vi "Center Scanner Tester.vi"(8 "Hight":u16, 9 "Width":u16, 10 "ImageIn":u8[][](array[numeric]), 11 "StartLine":u32) -> (1 "HorCenter":u16, 3 "ImgOut":u8[][](array[numeric]))   [LabVIEW 2015]
uses:
  <vilib>/Analysis/baseanly.llb/Mean (DBL).vi
  <vilib>/Analysis/NI_AALBase.lvlib
panel:
  out "mean 2":dbl format="%0.2f"
  out "mean":dbl format="%0.2f"
  out "ImageIn 2":u8[][](graph)
  out "ImgOut 2":u8[][](graph)
  out "max index(es) 2":i32
  out "element 2":dbl
  out "element":dbl
  out "max index(es)":i32
  out "size(s) 2":i32
  out "size(s)":i32
  out "Histogram Graph 2":T1(graph)
  out "Histogram Graph":T1(graph)
  out "Radiuses 2":i32[](graph)
  out "Centers 2":i32[](graph)
  out "Radiuses":i32[](graph)
  out "Centers":i32[](graph)
  in  "Delta":u32=2
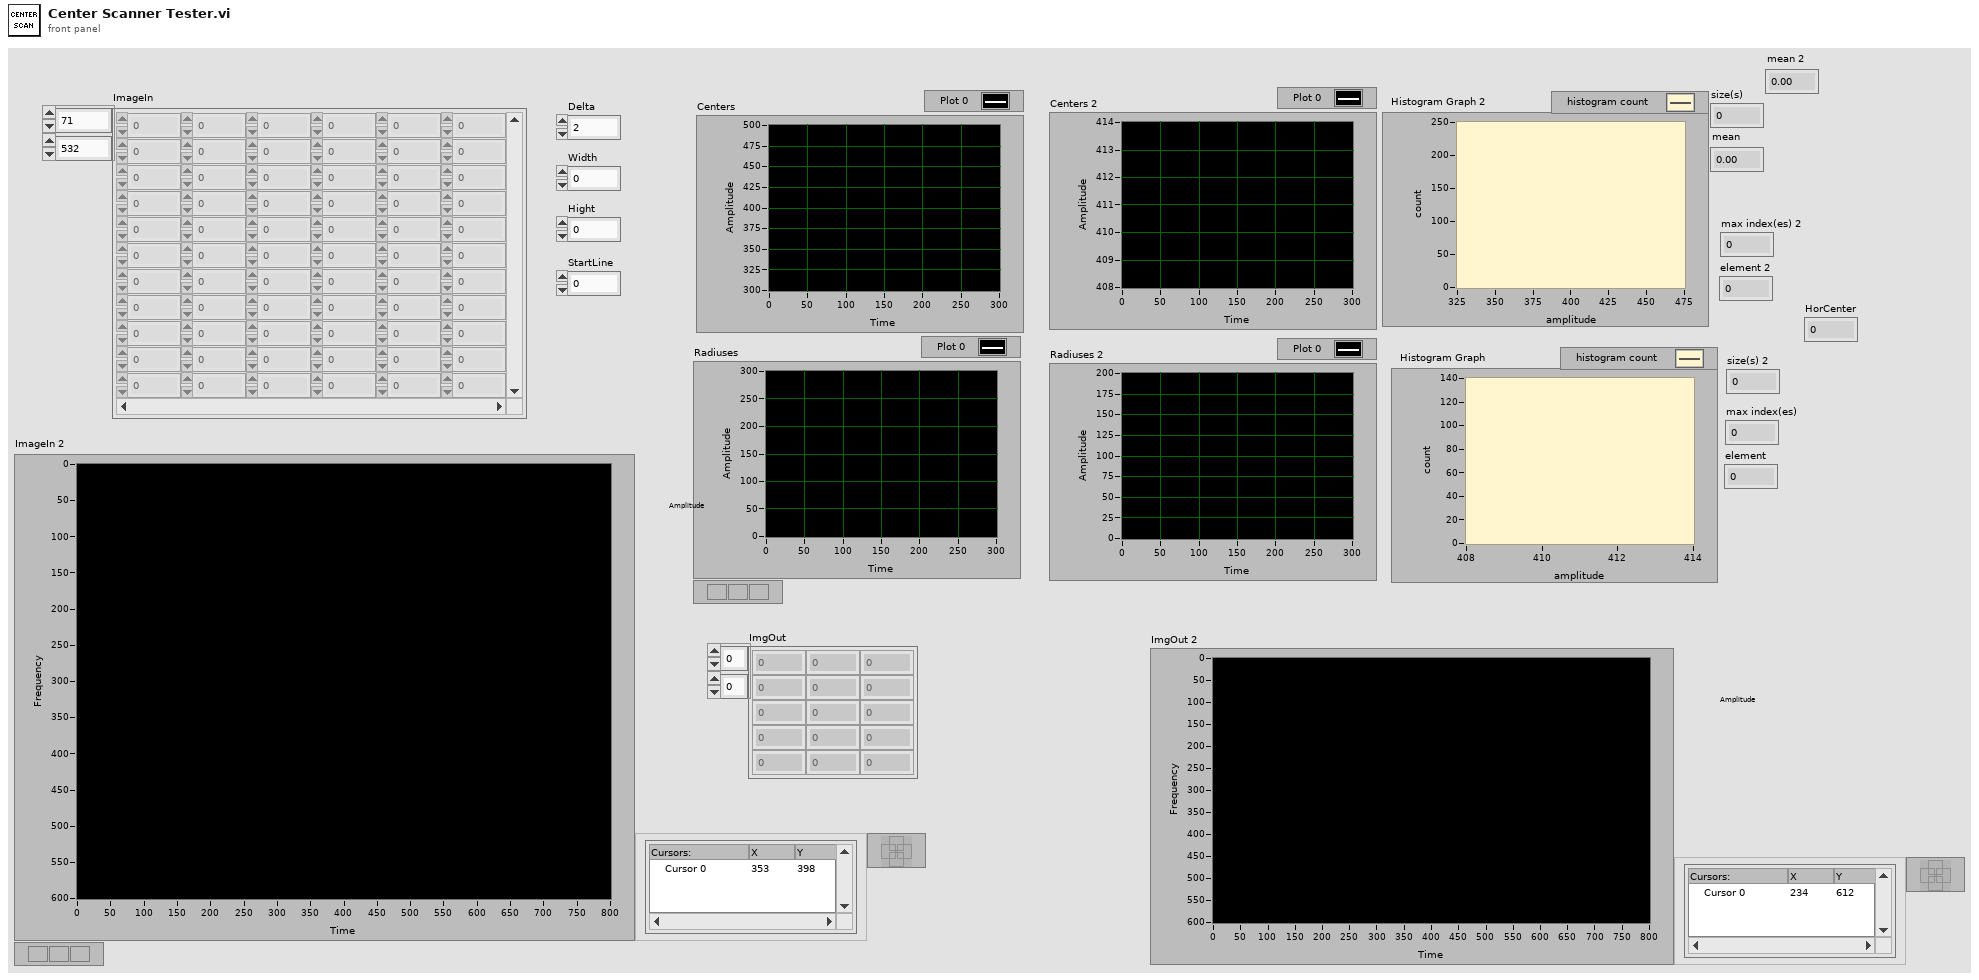
[diagram p1: front panel]
types:
  T1 = cluster{"X Values":dbl[], "Histogram: h(x)":i32[]}
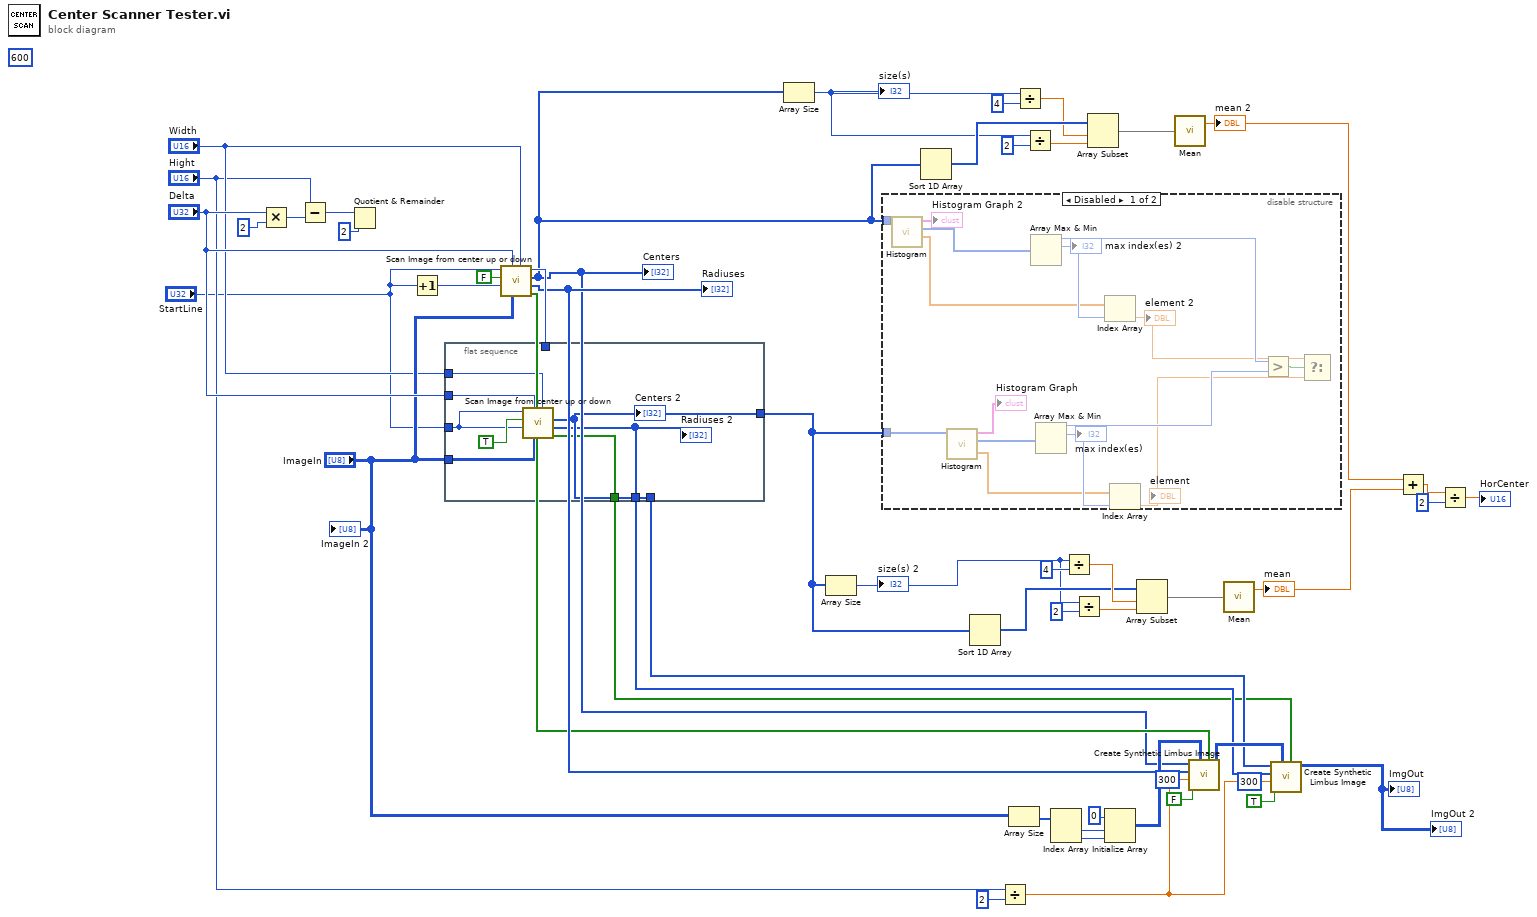
[diagram p0: block diagram]
diagram:
  (unwired) 300 ("Ofset")
  (unwired) 300 ("Ofset")
  (unwired) 600 ("element")
  n1 = Multiply(x="Delta", y=u8 2) -> (x*y=w46:u32)
  n2 = Subtract(x="Hight", y=w46) -> (x-y=w48:u32)
  n3 = Quotient & Remainder(x=w48, y=u32 2) -> ()  [unwired: 2 out]
  n4 = Increment(x="StartLine") -> (x+1=w42:u32)
  n5 = flat-sequence {
    tunnel: "ImageIn" -> [w57]
    tunnel: "Delta" -> [w55]
    tunnel: "StartLine" -> [w54]
    tunnel: w43 -> [_]
    tunnel: [w53] -> w7
    tunnel: [w53] -> w30
    tunnel: [w52] -> w31
    tunnel: "Width" -> [w51]
    tunnel: [w50] -> w24
    frame #0 {
      n6 = call "Scan Image from center up or down.vi"("Width"=w51, "ImageIn"=w57, "Delta"=w55, "StartLine"=w54, "UpDwn"=TRUE, "NoOfLines"=w54) -> ("OutLiars"=w50:bool[], "Radiuses"=w52:i32[], "Centers"=w53:i32[])  [unwired: 2 in, 1 out]
      "Centers 2" <- w53
      "Radiuses 2" <- w52
    }
  }
  n7 = call "Scan Image from center up or down.vi"("Width"="Width", "ImageIn"="ImageIn", "Delta"="Delta", "StartLine"=w42, "UpDwn"=FALSE, "NoOfLines"="StartLine") -> ("OutLiars"=w23:bool[], "Radiuses"=w34:i32[], "Centers"=w22:i32[], "Center"=w43:i32)  [unwired: 2 in]
  "Centers" <- w22
  "Radiuses" <- w34
  n8 = Array Size(array=w22) -> (size(s)=w17:i32)
  "size(s)" <- w17
  n9 = Array Size(array=w7) -> (size(s)=w8:i32)
  "size(s) 2" <- w8
  n10 = disable-structure shown="Disabled" {
    disable-tunnel: w22 -> [w59 _]
    disable-tunnel: w7 -> [w58 _]
    frame Disabled {
      n11 = call <vilib>:"Histogram.vi"("X"=w59) -> ("X Values"=w65:dbl[], "Histogram: h(x)"=w66:i32[], "Histogram Graph"=→"Histogram Graph 2":T1)  [unwired: 7 in, 1 out]
      n12 = call <vilib>:"Histogram.vi"("X"=w58) -> ("X Values"=w68:dbl[], "Histogram: h(x)"=w70:i32[], "Histogram Graph"=→"Histogram Graph":T1)  [unwired: 7 in, 1 out]
      n13 = Array Max & Min(array=w66) -> (max value=w64:i32, max index (indices)=w67:i32)  [unwired: 2 out]
      "max index(es) 2" <- w67
      n14 = Array Max & Min(array=w70) -> (max value=w63:i32, max index (indices)=w69:i32)  [unwired: 2 out]
      "max index(es)" <- w69
      n15 = Index Array(array=w65, index=w67) -> (element=w61:dbl)
      "element 2" <- w61
      n16 = Index Array(array=w68, index=w69) -> (element=w60:dbl)
      "element" <- w60
      n17 = Greater?(x=w64, y=w63) -> (0:w62:bool)
      n18 = Select(t=w61, s=w62, f=w60) -> ()  [unwired: 1 out]
    }
    frame Enabled {
    }
  }
  n19 = Sort 1D Array(array=w22) -> (sorted array=w20:i32[])
  n20 = Sort 1D Array(array=w7) -> (sorted array=w10:i32[])
  n21 = Divide(x="Hight", y=u16 2) -> (x/y=w25:dbl)
  n22 = Array Size(array="ImageIn") -> (size(s)=w41:i32[])
  n23 = Divide(x=w17, y=4) -> (x/y=w18:dbl)
  n24 = Divide(x=w17, y=2) -> (x/y=w16:dbl)
  n25 = Index Array(array=w41) -> (element #1=w40:i32, element #2=w39:i32)  [unwired: 2 in]
  n26 = Divide(x=w8, y=4) -> (x/y=w12:dbl)
  n27 = Divide(x=w8, y=2) -> (x/y=w13:dbl)
  n28 = Array Subset(array=w20, index=w18, length=w16) -> (w15:i32[])
  n29 = Initialize Array(u8 0, w40, w39) -> (w37:u8[][])
  n30 = Array Subset(array=w10, index=w12, length=w13) -> (w14:i32[])
  n31 = call-poly <vilib>:"Mean.vi"("X"=w15) -> ("mean"=w6:dbl)  [unwired: 1 out]
  "mean 2" <- w6
  n32 = call "Create Synthetic Limbus Image.vi"("OutLiars"=w23, "Array in"=w37, "Direction"=FALSE, "Ofset"=w25, "Radiuse"=w34, "Centers"=w22) -> ("Array out"=w36:u8[][])  [unwired: 5 in]
  n33 = call-poly <vilib>:"Mean.vi"("X"=w14) -> ("mean"=w5:dbl)  [unwired: 1 out]
  "mean" <- w5
  n34 = call "Create Synthetic Limbus Image.vi"("OutLiars"=w24, "Array in"=w36, "Direction"=TRUE, "Ofset"=w25, "Radiuse"=w31, "Centers"=w30) -> ("Array out"=→"ImgOut" →"ImgOut 2":u8[][])  [unwired: 5 in]
  n35 = Add(x=w6, y=w5) -> (x+y=w3:dbl)
  n36 = Divide(x=w3, y=2) -> (x/y=→"HorCenter":dbl)
  "ImageIn 2" <- "ImageIn"
